vi "Uninitalized Shift Registers.vi"() -> ()   [LabVIEW 2015]
panel:
  out "Answer 2?":dbl
  out "Answer 1?":dbl
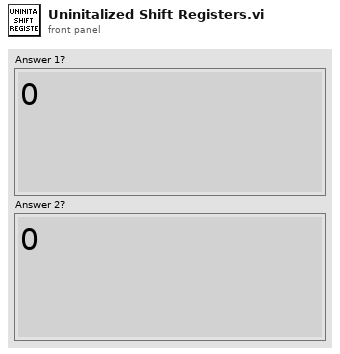
[diagram p1: front panel]
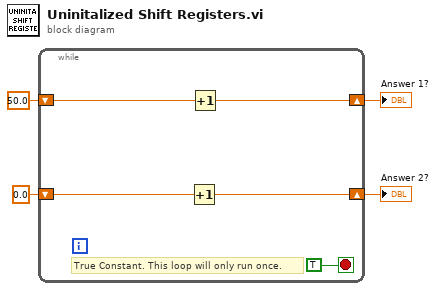
[diagram p0: block diagram]
diagram:
  n1 = while {
    shift-right: [w8] -> w4
    shift-left: 50.0 -> [w9]
    shift-right: [w6] -> w2
    shift-left: 0.0 -> [w5]
    stop <- TRUE stop-if-true
    # "True Constant. This loop will only run once."
    n2 = Increment(x=w5) -> (x+1=w6:dbl)
    n3 = Increment(x=w9) -> (x+1=w8:dbl)
  }
  "Answer 1?" <- w4
  "Answer 2?" <- w2
